vi "CPP_WhiteNoisePlayer.vi"() -> ()   [LabVIEW 2011]
uses:
  <vilib>/sound/lvsound.llb/Sound Format.ctl
  <vilib>/Analysis/NI_AALBase.lvlib
panel:
  in  "Duration":dbl(slide) scale=0.0..10.0
  in  "Amplitude":dbl(knob) scale=0.0..11.0
  out "error out":errorcluster
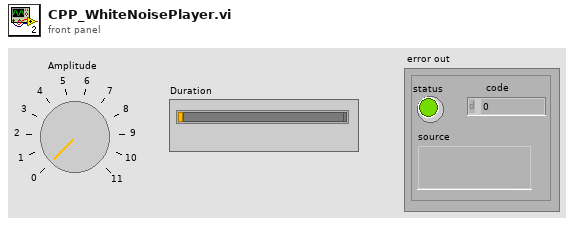
[diagram p1: front panel]
types:
  T1 = typedef "Sound Format.ctl" = cluster{"sound quality":enum16{"mono", "stereo"}, "rate":enum16{"11025", "22050", "44100", "8000"}, "bits per sample":enum16{"8 bit", "16 bit"}}
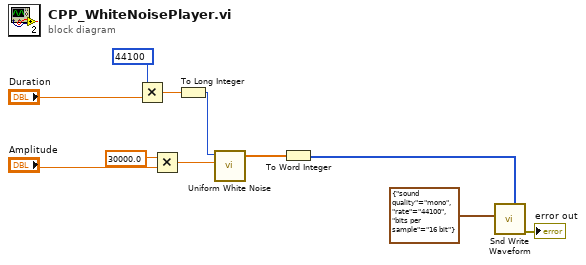
[diagram p0: block diagram]
diagram:
  n1 = Multiply(x=44100 ("samples"), y="Duration") -> (x*y=w3:dbl)
  n2 = Multiply(x=30000.0, y="Amplitude") -> (x*y=w7:dbl)
  n3 = To Long Integer(number=w3) -> (32bit integer=w1:i32)
  n4 = call <vilib>:"Uniform White Noise.vi"("amplitude"=w7, "samples"=w1) -> ("uniform white noise"=w8:dbl[])  [unwired: 8 in, 1 out]
  n5 = To Word Integer(number=w8) -> (16bit integer=w9:i16[])
  n6 = call <vilib>:"Snd Write Waveform.vi"("mono 16-bit"=w9, "sound format"=T1 {"sound quality"=enum."mono", "rate"=enum."44100", "bits per sample"=enum."16 bit"}) -> ("error out"=→"error out":errorcluster)  [unwired: 9 in]
